vi "FPG10.vi"() -> ()   [LabVIEW 2021]
uses:
  <vilib>/rvi/Emulation/niFpgaGetClockAttributes.vi
  <vilib>/rvi/Emulation/niFpgaSctlEmulationGetInTimedLoop.vi
  <vilib>/rvi/Emulation/niFpgaEmulationReportErrorSimple.vi
  <vilib>/rvi/eio/common/nirviEmuTemplateMethod_errors.vi
  <vilib>/rvi/Emulation/niFpgaCriticalErrorInLSC.vi
  <vilib>/eio/EIONode/EIONode.xnode
panel:
  out "ConnectorC/AI1":i16
  out "ConnectorB/DIO13":bool
  out "ConnectorB/DIO4":bool
  out "ConnectorB/DIO3":bool
  out "ConnectorB/DIO2":bool
  out "ConnectorB/DIO1":bool
  out "ConnectorB/DIO0":bool
  out "ConnectorC/AI0":i16
  out "ConnectorA/DIO13":bool
  out "ConnectorA/DIO4":bool
  out "ConnectorA/DIO3":bool
  out "ConnectorA/DIO2":bool
  out "ConnectorA/DIO1":bool
  out "ConnectorA/DIO0":bool
  in  "stop":bool
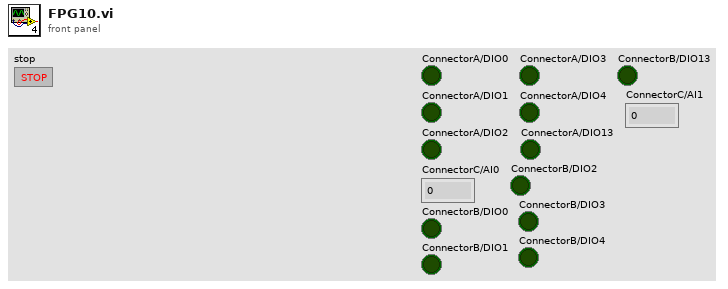
[diagram p1: front panel]
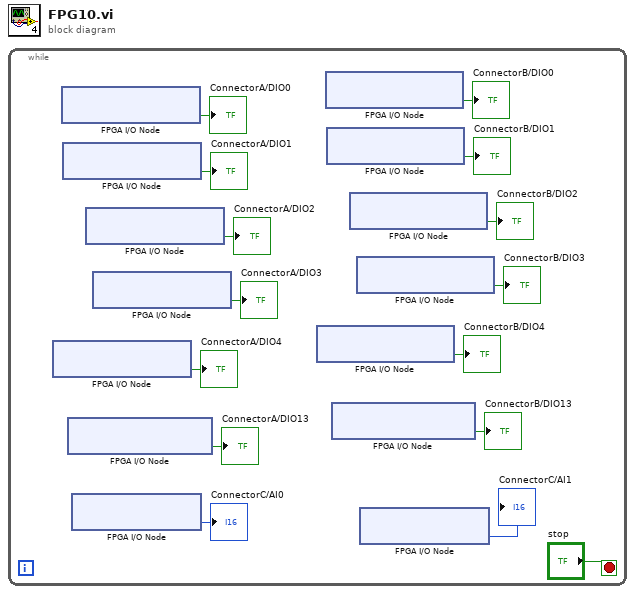
[diagram p0: block diagram]
diagram:
  n1 = while {
    stop <- "stop" stop-if-true
    n2 = xnode "FPGA I/O Node"() -> ("ConnectorA/DIO4"=→"ConnectorA/DIO4":bool)  [unwired: 1 in, 1 out]
    n3 = xnode "FPGA I/O Node"() -> ("ConnectorA/DIO0"=→"ConnectorA/DIO0":bool)  [unwired: 1 in, 1 out]
    n4 = xnode "FPGA I/O Node"() -> ("ConnectorA/DIO1"=→"ConnectorA/DIO1":bool)  [unwired: 1 in, 1 out]
    n5 = xnode "FPGA I/O Node"() -> ("ConnectorA/DIO13"=→"ConnectorA/DIO13":bool)  [unwired: 1 in, 1 out]
    n6 = xnode "FPGA I/O Node"() -> ("ConnectorC/AI0"=→"ConnectorC/AI0":i16)  [unwired: 1 in, 1 out]
    n7 = xnode "FPGA I/O Node"() -> ("ConnectorA/DIO2"=→"ConnectorA/DIO2":bool)  [unwired: 1 in, 1 out]
    n8 = xnode "FPGA I/O Node"() -> ("ConnectorA/DIO3"=→"ConnectorA/DIO3":bool)  [unwired: 1 in, 1 out]
    n9 = xnode "FPGA I/O Node"() -> ("ConnectorB/DIO4"=→"ConnectorB/DIO4":bool)  [unwired: 1 in, 1 out]
    n10 = xnode "FPGA I/O Node"() -> ("ConnectorB/DIO0"=→"ConnectorB/DIO0":bool)  [unwired: 1 in, 1 out]
    n11 = xnode "FPGA I/O Node"() -> ("ConnectorB/DIO1"=→"ConnectorB/DIO1":bool)  [unwired: 1 in, 1 out]
    n12 = xnode "FPGA I/O Node"() -> ("ConnectorB/DIO13"=→"ConnectorB/DIO13":bool)  [unwired: 1 in, 1 out]
    n13 = xnode "FPGA I/O Node"() -> ("ConnectorB/DIO2"=→"ConnectorB/DIO2":bool)  [unwired: 1 in, 1 out]
    n14 = xnode "FPGA I/O Node"() -> ("ConnectorB/DIO3"=→"ConnectorB/DIO3":bool)  [unwired: 1 in, 1 out]
    n15 = xnode "FPGA I/O Node"() -> ("ConnectorC/AI1"=→"ConnectorC/AI1":i16)  [unwired: 1 in, 1 out]
  }
